vi "Set Voltage.vi"(8 "error in":errorcluster, 10 "V":dbl, 11 "Session HVPS in":refnum<class "Session HVPS.lvclass">) -> (0 "error out":errorcluster, 3 "Session HVPS out":refnum<class "Session HVPS.lvclass">)   [LabVIEW 2014, in "Session HVPS.lvclass"]
uses:
  Session HVPS.lvclass
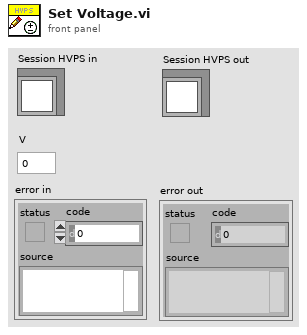
[diagram p1: front panel]
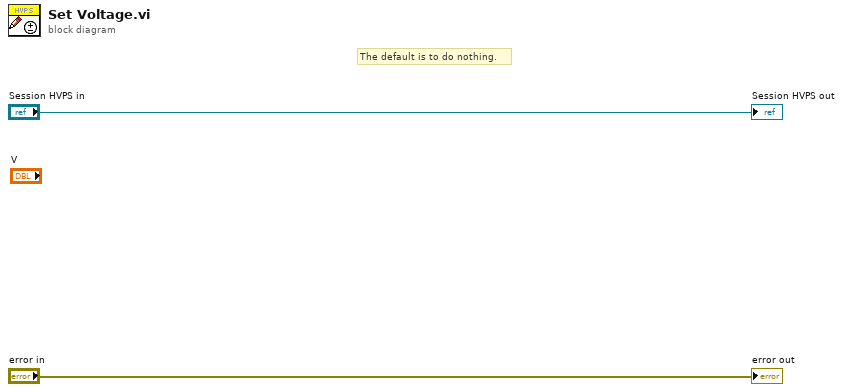
[diagram p0: block diagram]
diagram:
  # "The default is to do nothing."
  "error out" <- "error in"
  "Session HVPS out" <- "Session HVPS in"
